vi "p2.vi"() -> ()   [LabVIEW 2025, in "d2.lvlib"]
uses:
  d2.lvlib
  a064d2ae-a9d4-4372-b67c-8354b34c0d52.vi
  AOC/AOC.lvlib
panel:
  in  "Example":string="11-22,95-115,998-1012,1188511880-1188511890,222220-222224,\n1698522-1698528,446443-446449,38593856-38593862,565653-565659,\n824824821-824824827,2121212118-2121212124"
  in  "Example 2":bool
  out "Answer":i64=10624
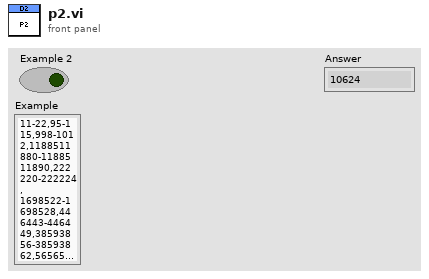
[diagram p1: front panel]
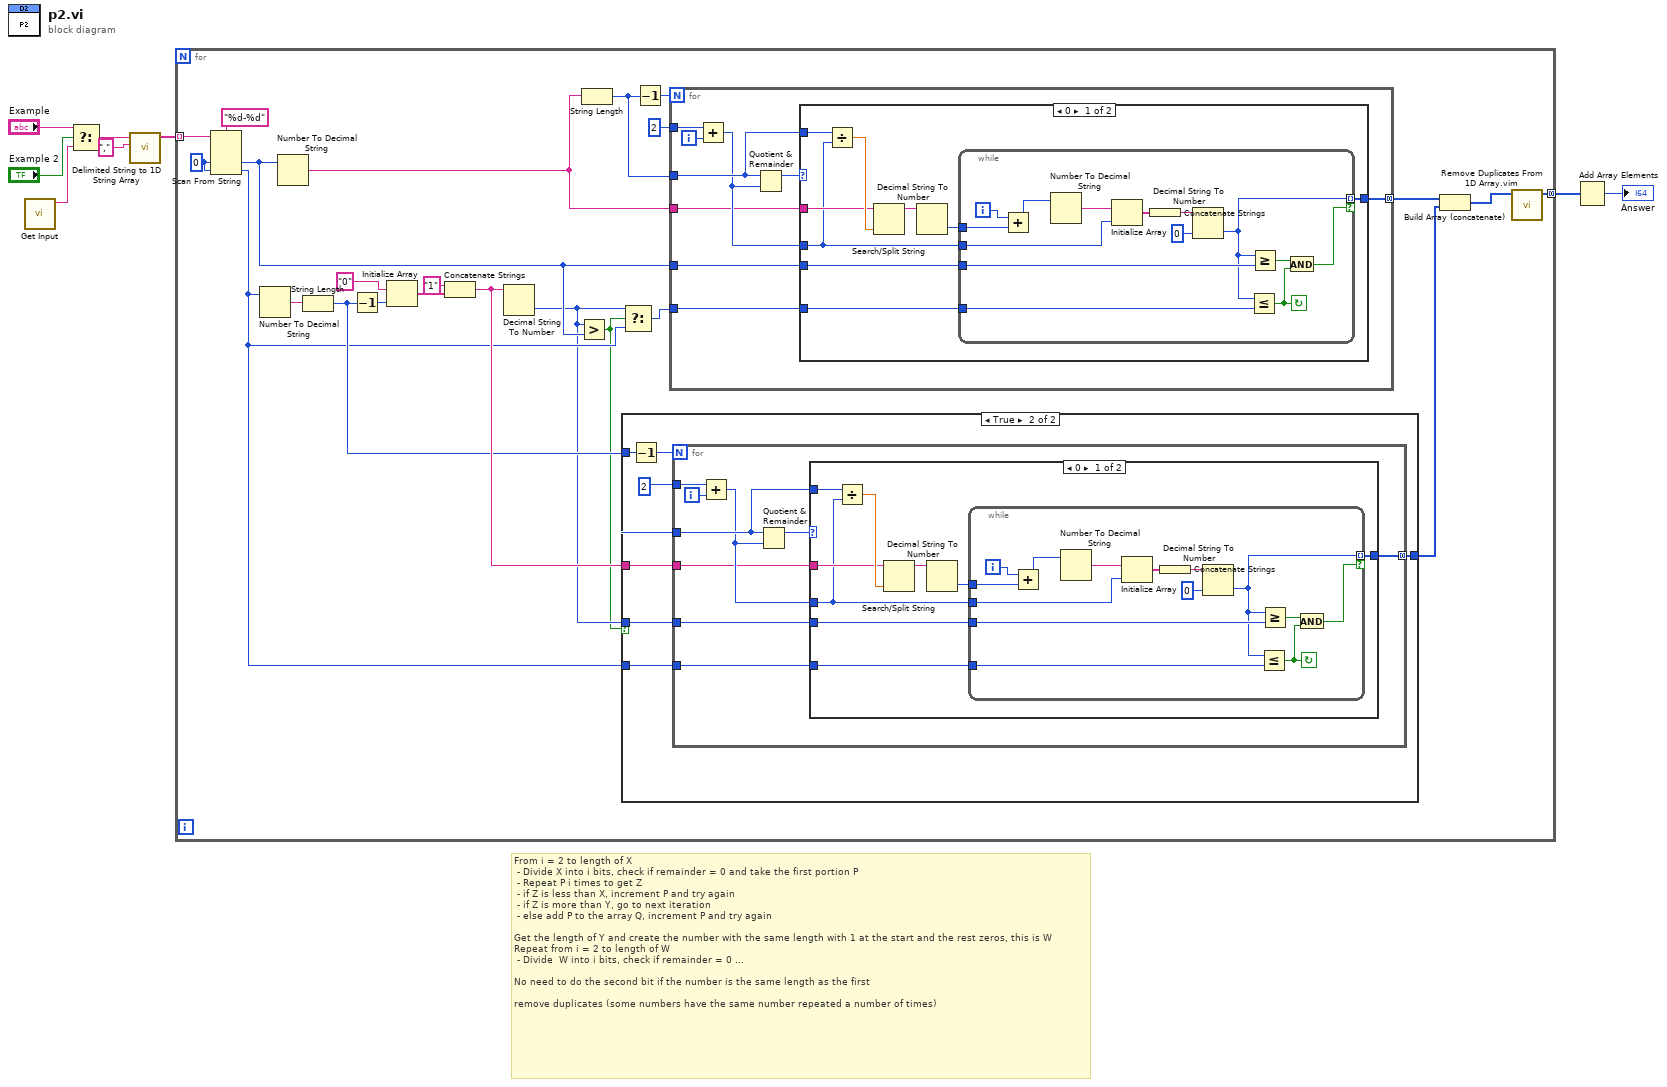
[diagram p0: block diagram]
diagram:
  # "From i = 2 to length of X\n - Divide X into i bits, check if remainder = 0 and take the first portion P \n - Repeat P i times to get Z\n - if Z is less than X, increment P and try again\n - if Z is more than Y, go to next iteration\n - else add P to the array Q, increment P and try again\n\nGet the length of Y and create the number with the same length with 1 at the start and the rest zeros, this is W\nRepeat from i = 2 to length of W\n - Divide  W into i bits, check if remainder = 0 ...\n\nNo need to do the second bit if the number is the same length as the first\n\nremove duplicates (some numbers have the same number repeated a number of times)"
  n1 = call "Get Input.vi"() -> ("Input"=w8:string)  [unwired: 11 in]
  n2 = Select(t="Example", s="Example 2", f=w8) -> (s? t:f=w7:string)
  n3 = call <vilib>:"Delimited String to 1D String Array.vi"("delimiter"=",", "delimited string"=w7) -> ("string array"=w2:string[])  [unwired: 9 in]
  n4 = for {
    tunnel: w2 -> [w31] mode=indexing
    tunnel: [w15] -> w1 mode=concatenating
    w29 = i64 0 ("default value 14")
    n5 = Scan From String(format string="%d-%d", input string=w31, default 1=w29, default 2=w29) -> (output 1=w14:i64, output 2=w13:i64)  [unwired: 2 in, 3 out]
    n6 = Number To Decimal String(number=w13) -> (decimal integer string=w24:string)  [unwired: 1 in]
    n7 = Number To Decimal String(number=w14) -> (decimal integer string=w25:string)  [unwired: 1 in]
    n8 = String Length(string=w24) -> (length=w18:i32)
    n9 = Decrement(x=w18) -> (x-1=w23:i32)
    n10 = Initialize Array("0" ("element"), w23) -> (w21:string[])
    n11 = Concatenate Strings("1" ("string"), w21) -> (w19:string)
    n12 = Decimal String To Number(string=w19) -> (number=w12:i32)  [unwired: 2 in, 1 out]
    n13 = Greater?(x=w12, y=w14) -> (0:w10:bool)
    n14 = String Length(string=w25) -> (length=w26:i32)
    n15 = case shown="True" w10 {
      tunnel: w19 -> [_ w68]
      tunnel: w18 -> [_ w67]
      tunnel: [_ w66] -> w17
      tunnel: w12 -> [_ w65]
      tunnel: w13 -> [_ w64]
      frame False {
      }
      frame True {
        n16 = Decrement(x=w67) -> (x-1=w70:i32)
        n17 = for {
          N: w70 -> [_]
          tunnel: 2 ("y") -> [w78]
          tunnel: w67 -> [w76]
          tunnel: w68 -> [w74]
          tunnel: w65 -> [w73]
          tunnel: w64 -> [w72]
          tunnel: [w71] -> w66 mode=concatenating
          i -> [w79]
          n18 = Add(x=w78, y=w79) -> (x+y=w75:i32)
          n19 = Quotient & Remainder(x=w76, y=w75) -> (x-y*floor(x/y)=w77:i32)  [unwired: 1 out]
          n20 = case shown="0" w77 {
            tunnel: w76 -> [w88 _]
            tunnel: w75 -> [w85 _]
            tunnel: w74 -> [w86 _]
            tunnel: w73 -> [w84 _]
            tunnel: w72 -> [w83 _]
            tunnel: [w82 _] -> w71
            frame 0 {
              n21 = Divide(x=w88, y=w85) -> (x/y=w87:dbl)
              n22 = Search/Split String(string=w86, offset (0)=w87) -> (substring before match=w81:string)  [unwired: 1 in, 2 out]
              n23 = Decimal String To Number(string=w81) -> (number=w80:i32)  [unwired: 2 in, 1 out]
              n24 = while {
                tunnel: w85 -> [w102]
                tunnel: w84 -> [w98]
                tunnel: w83 -> [w97]
                tunnel: [w96] -> w82 mode=indexing if=w92
                tunnel: w80 -> [w94]
                i -> [w89]
                stop <- w91 continue-if-true
                n25 = Add(x=w89, y=w94) -> (x+y=w90:i32)
                n26 = Number To Decimal String(number=w90) -> (decimal integer string=w93:string)  [unwired: 1 in]
                n27 = Initialize Array(w93, w102) -> (w101:string[])
                n28 = Concatenate Strings(w101) -> (w100:string)
                n29 = Decimal String To Number(string=w100, default (0L)=i64 0 ("default (0 I32)")) -> (number=w96:i64)  [unwired: 1 in, 1 out]
                n30 = Less Or Equal?(x=w96, y=w97) -> (x <= y?=w91:bool)
                n31 = Greater Or Equal?(x=w96, y=w98) -> (x >= y?=w95:bool)
                n32 = And(x=w95, y=w91) -> (x .and. y?=w92:bool)
              }
            }
            frame Default {
            }
          }
        }
      }
    }
    n33 = Select(t=w12, s=w10, f=w13) -> (s? t:f=w11:i64)
    n34 = Decrement(x=w26) -> (x-1=w28:i32)
    n35 = for {
      N: w28 -> [_]
      tunnel: 2 ("y") -> [w39]
      tunnel: w26 -> [w37]
      tunnel: w25 -> [w35]
      tunnel: w14 -> [w34]
      tunnel: w11 -> [w33]
      tunnel: [w32] -> w9 mode=concatenating
      i -> [w40]
      n36 = Add(x=w39, y=w40) -> (x+y=w36:i32)
      n37 = Quotient & Remainder(x=w37, y=w36) -> (x-y*floor(x/y)=w38:i32)  [unwired: 1 out]
      n38 = case shown="0" w38 {
        tunnel: w37 -> [w49 _]
        tunnel: w36 -> [w46 _]
        tunnel: w35 -> [w47 _]
        tunnel: w34 -> [w45 _]
        tunnel: w33 -> [w44 _]
        tunnel: [w43 _] -> w32
        frame 0 {
          n39 = Divide(x=w49, y=w46) -> (x/y=w48:dbl)
          n40 = Search/Split String(string=w47, offset (0)=w48) -> (substring before match=w42:string)  [unwired: 1 in, 2 out]
          n41 = Decimal String To Number(string=w42) -> (number=w41:i32)  [unwired: 2 in, 1 out]
          n42 = while {
            tunnel: w46 -> [w63]
            tunnel: w45 -> [w59]
            tunnel: w44 -> [w58]
            tunnel: [w57] -> w43 mode=indexing if=w53
            tunnel: w41 -> [w55]
            i -> [w50]
            stop <- w52 continue-if-true
            n43 = Add(x=w50, y=w55) -> (x+y=w51:i32)
            n44 = Number To Decimal String(number=w51) -> (decimal integer string=w54:string)  [unwired: 1 in]
            n45 = Initialize Array(w54, w63) -> (w62:string[])
            n46 = Concatenate Strings(w62) -> (w61:string)
            n47 = Decimal String To Number(string=w61, default (0L)=i64 0 ("default (0 I32)")) -> (number=w57:i64)  [unwired: 1 in, 1 out]
            n48 = Less Or Equal?(x=w57, y=w58) -> (x <= y?=w52:bool)
            n49 = Greater Or Equal?(x=w57, y=w59) -> (x >= y?=w56:bool)
            n50 = And(x=w56, y=w52) -> (x .and. y?=w53:bool)
          }
        }
        frame Default {
        }
      }
    }
    n51 = Build Array (concatenate)(w9, w17) -> (w16:i64[])
    n52 = call "Remove Duplicates From 1D Array.vim"("array"=w16) -> ("array with duplicates removed"=w15:i64[])  [unwired: 10 in]
  }
  n53 = Add Array Elements(numeric array=w1) -> (sum=→"Answer":i64)
